vi "vis_acq_disassemble_everyFrame.vi"(5 "Stop (F)":bool, 7 "error in":errorcluster) -> (20 "Image Out":T1(plugin-control), 21 "All Image Buffers Out":T1[](array[typedef]), 26 "Stopped":bool, 27 "error out":errorcluster)   [LabVIEW 2013]
doc: "Creates, and edits acquisitions using the NI Vision Acquisition Express VI.\n\nThe NI Vision Acquisition Wizard is launched by placing the Express VI on the block diagram. Select an acquisition source and configure an acquisition using NI-IMAQ, NI-IMAQdx, or simulate an acquisition by reading an AVI or image files from a folder. After an acquisition is configured, select controls and indicators to be able to programmatically set in LabVIEW. Double-click the Vision Acquisition Express VI to edit the acquisition.\n\nNote: Any images created by the Express VI need to be disposed after use. Use the IMAQ Dispose.vi to cleanup the images output by the Express VI when they are no longer needed."
uses:
  <vilib>/vision/Image Controls.llb/IMAQ Image.ctl
  <vilib>/vision/driver/IMAQdx.llb/IMAQdx Buffer Number Mode.ctl
  <vilib>/vision/driver/Vision Acquisition Express Utility VIs.llb/Vision Acquisition Path Convert (String).vi
  <vilib>/vision/driver/NI_Vision_Acquisition_Software.lvlib
  <resource>/objmgr/imaqdx.rc
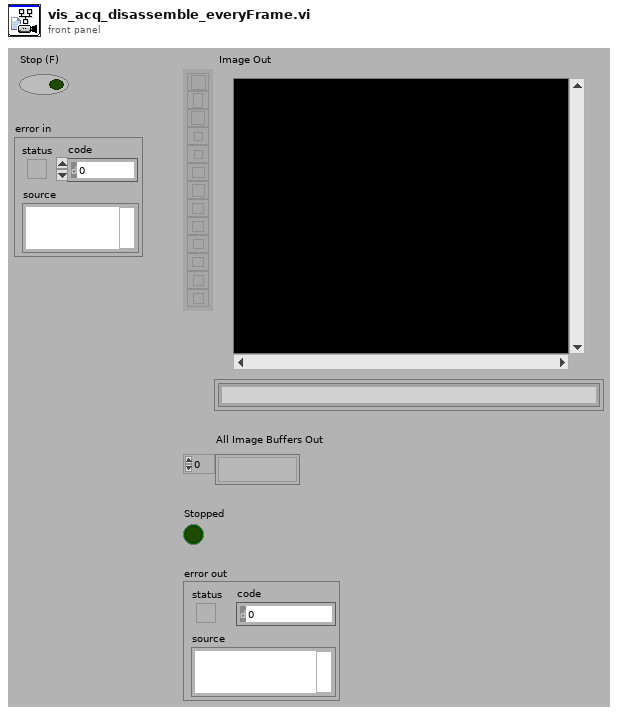
[diagram p1: front panel]
types:
  T1 = typedef "IMAQ Image.ctl" = refnum<image>
  T2 = typedef "NI_Vision_Acquisition_Software.lvlib/IMAQdx Buffer Number Mode.ctl" = enum32{"Next", "Last", "Buffer Number"}
  T3 = typedef "IMAQdx.ctl" = refnum<k21>
  T4 = cluster{"File Type":string, "Quality":u32, "Compress":bool, "Lossless":bool, "Ratio":sgl, "Codec":string, "Frame Rate":u32, "Limit Frames":bool, "Max Frames":u32}
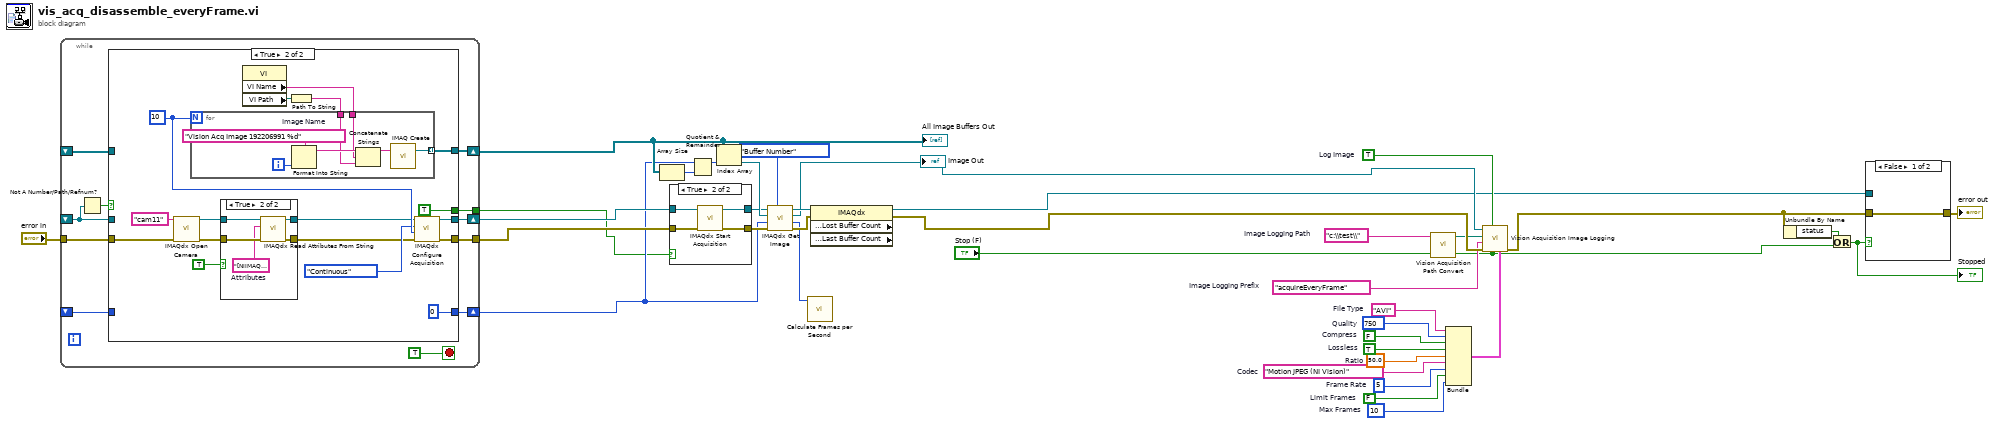
[diagram p0: block diagram]
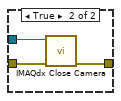
[diagram p2: hidden frame]
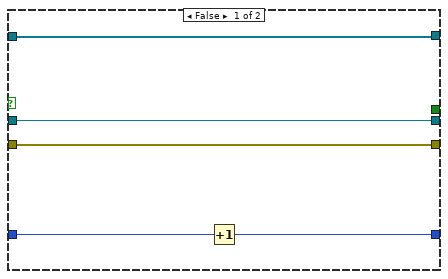
[diagram p4: hidden frame]
diagram:
  w6 = "c:\\test\\"  # Image Logging Path
  w9 = TRUE  # Log Image
  w20 = "acquireEveryFrame"  # Image Logging Prefix
  w15 = sgl 50.0  # Ratio
  w16 = TRUE  # Lossless
  w17 = FALSE  # Compress
  w18 = u32 750  # Quality
  w14 = "Motion JPEG (NI Vision)"  # Codec
  w13 = u32 5  # Frame Rate
  w11 = u32 10  # Max Frames
  w12 = FALSE  # Limit Frames
  w19 = "AVI"  # File Type
  n1 = while {
    shift-right: [w48] -> w28
    shift-left: _ -> [w40]
    tunnel: [w47] -> w36
    tunnel: "error in" -> [w46]
    shift-right: [w44] -> w32
    shift-left: _ -> [w43]
    shift-right: [w42] -> w25
    shift-left: _ -> [w41]
    tunnel: [w38] -> w24
    stop <- TRUE stop-if-true
    n2 = Not A Number/Path/Refnum?(number/path/refnum=w40) -> (NaN/Path/Refnum?=w39:bool)
    n3 = case shown="True" w39 {
      tunnel: [w53 w68] -> w48
      tunnel: w40 -> [w53 _]
      tunnel: [w52 w67] -> w47
      tunnel: w46 -> [w52 w70]
      tunnel: [w51 w66] -> w44
      tunnel: w43 -> [w51 _]
      tunnel: [w49 0] -> w42
      tunnel: w41 -> [w50 _]
      tunnel: [_ TRUE] -> w38
      frame False {
        n4 = Increment(x=w50) -> (x+1=w49:i32)
      }
      frame True {
        w65 = u32 10 ("Number of Image Buffers")
        n5 = call <vilib>:"IMAQdx Open Camera.vi"("error in"=w70, "Session In"="cam11" ("Interface Name")) -> ("error out"=w58:errorcluster, "Session Out"=w59:T3)  [unwired: 1 in, 7 out]
        n6 = case shown="True" TRUE ("Init Attributes") {
          tunnel: w59 -> [w72 w77]
          tunnel: w58 -> [w71 w76]
          tunnel: [w72 w74] -> w57
          tunnel: [w71 w73] -> w56
          frame False {
          }
          frame True {
            w75 = "[NIIMAQ_HEADER]\nType = 2\nVersion = 8\n\n[CAMERA_DATA]\nAcquisitionAttributes::Bayer::Algorithm = \"Bilinear\"\nAcquisitionAttributes::Bayer::GainB = \"1\"\nAcquisitionAttributes::Bayer::GainG = \"1\"\nAcquisitionAttributes::Bayer::GainR = \"1\"\nAcquisitionAttributes::Bayer::Pattern = \"Use hardware value\"\nAcquisitionAttributes::BitsPerPixel = \"Use hardware value\"\nAcquisitionAttributes::IgnoreFirstFrame = \"false\"\nAcquisitionAttributes::ImageDecoderCopyMode = \"Auto\"\nAcquisitionAttributes::OutputImageType = \"Auto\"\nAcquisitionAttributes::OverwriteMode = \"Get Newest\"\nAcquisitionAttributes::PixelSignedness = \"Use hardware value\"\nAcquisitionAttributes::ReceiveTimestampMode = \"None\"\nAcquisitionAttributes::ShiftPixelBits = \"false\"\nAcquisitionAttributes::SwapPixelBytes = \"false\"\nAcquisitionAttributes::Timeout = \"5000\"\nAcquisitionAttributes::VerticalMirror = \"false\"\nAcquisitionAttributes::VideoMode = \"1280x720 RGB24 30.00fps\"\nCameraAttributes::BacklightCompensation::Mode = \"Manual\"\nCameraAttributes::BacklightCompensation::Value = \"false\"\nCameraAttributes::Brightness::Mode = \"Manual\"\nCameraAttributes::Brightness::Value = \"133\"\nCameraAttributes::Contrast::Mode = \"Manual\"\nCameraAttributes::Contrast::Value = \"0.050000000000000003\"\nCameraAttributes::Exposure::Mode = \"Auto\"\nCameraAttributes::Pan::Mode = \"Manual\"\nCameraAttributes::Pan::Value = \"0\"\nCameraAttributes::Saturation::Mode = \"Manual\"\nCameraAttributes::Saturation::Value = \"83\"\nCameraAttributes::Sharpness::Mode = \"Manual\"\nCameraAttributes::Sharpness::Value = \"1\"\nCameraAttributes::Tilt::Mode = \"Manual\"\nCameraAttributes::Tilt::Value = \"0\"\nCameraAttributes::WhiteBalance::Mode = \"Auto\"\nCameraAttributes::Zoom::Mode = \"Manual\"\nCameraAttributes::Zoom::Value = \"0\"\n"  # Attributes
            n7 = call <vilib>:"IMAQdx Read Attributes From String.vi"("error in"=w76, "Attributes String In"=w75, "Session In"=w77) -> ("error out"=w73:errorcluster, "Session Out"=w74:T3)  [unwired: 7 out]
          }
        }
        n8 = property class="VI"() -> ("VI Name"=w61:string, "VI Path"=w62:path)  [unwired: 2 in, 2 out]
        n9 = Path To String(path=w62) -> (string=w60:string)
        n10 = for "For Loop_template0" {
          N: w65 -> [_]
          tunnel: [w84] -> w66 mode=indexing
          tunnel: w61 -> [w79]
          tunnel: w60 -> [w78]
          i -> [w83]
          w82 = "Vision Acq Image 192206991 %d"  # Image Name
          n11 = Format Into String(format string=w82, w83) -> (resulting string=w81:string)  [unwired: 2 in, 1 out]
          n12 = Concatenate Strings(w81, w79, w78) -> (w80:string)
          n13 = call "IMAQ Create"("Image Name"=w80) -> ("New Image"=w84:T1)  [unwired: 3 in, 2 out]
        }
        n14 = call <vilib>:"IMAQdx Configure Acquisition.vi"("error in"=w56, "Number of Buffers"=w65, "Continuous?"=enum32{"One Shot", "Continuous"}."Continuous" ("Mode"), "Session In"=w57) -> ("error out"=w67:errorcluster, "Session Out"=w68:T3)  [unwired: 6 out]
      }
    }
  }
  "All Image Buffers Out" <- w32
  n15 = Array Size(array=w32) -> (size(s)=w33:i32)
  n16 = case shown="True" w24 {
    tunnel: w28 -> [w86 w90]
    tunnel: w36 -> [w85 w89]
    tunnel: [w85 w88] -> w26
    tunnel: [w86 w87] -> w27
    frame False {
    }
    frame True {
      n17 = call <vilib>:"IMAQdx Start Acquisition.vi"("error in"=w89, "Session In"=w90) -> ("error out"=w88:errorcluster, "Session Out"=w87:T3)  [unwired: 8 out]
    }
  }
  n18 = Quotient & Remainder(x=w25, y=w33) -> (x-y*floor(x/y)=w31:i32)  [unwired: 1 out]
  n19 = Index Array(array=w32, index=w31) -> (element=w30:T1)
  n20 = call <vilib>:"IMAQdx Get Image.vi"("Buffer Number Mode (Next)"=IMAQdx_Buffer_Number_Mode."Buffer Number", "error in"=w26, "Buffer Number In"=w25, "Image In"=w30, "Session In"=w27) -> ("error out"=w34:errorcluster, "Buffer Number Out"=w23:u32, "Image Out"=w21:T1, "Session Out"=w35:T3)  [unwired: 3 out]
  "Image Out" <- w21
  n21 = call <vilib>:"Calculate Frames per Second.vi"("Buffer Number"=w23) -> ()  [unwired: 2 in, 9 out]
  n22 = property class="IMAQdx" props=["Status Information:Lost Buffer Count", "Status Information:Last Buffer Count"](reference=w35, error in=w34) -> (reference out=w5:T3, error out=w29:errorcluster)  [unwired: 2 out]
  n23 = call-poly <vilib>:"Vision Acquisition Path Convert.vi"("Path In"=w6) -> ("Path Out"=w7:path)  [unwired: 10 in]
  n24 = Bundle("File Type"=w19, "Quality"=w18, "Compress"=w17, "Lossless"=w16, "Ratio"=w15, "Codec"=w14, "Frame Rate"=w13, "Limit Frames"=w12, "Max Frames"=w11) -> (w8:T4)  [unwired: 1 out]
  n25 = call <vilib>:"Vision Acquisition Image Logging.vi"("File Settings"=w8, "Close"="Stop (F)", "Log Image"=w9, "error in (no error)"=w29, "Image Logging Prefix"=w20, "Image Logging Path"=w7, "Image In"=w21) -> ("error out"=w10:errorcluster)  [unwired: 4 out]
  n26 = Unbundle By Name(w10) -> ("status"=w1:bool)
  n27 = Or(x=w1, y="Stop (F)") -> (x .or. y?=w2:bool)
  "Stopped" <- w2
  n28 = case "Case Structure_template1" shown="False" w2 {
    tunnel: [w91 w93] -> w4
    tunnel: w10 -> [w91 w94]
    tunnel: w5 -> [_ w92]
    frame False {
    }
    frame True {
      n29 = call <vilib>:"IMAQdx Close Camera.vi"("error in"=w94, "Session In"=w92) -> ("error out"=w93:errorcluster)  [unwired: 9 out]
    }
  }
  "error out" <- w4
